vi "scale raw data.vi"(6 "ch3":waveform(dbl), 7 "Signal scaling control":T2={"Iin ripple gain"=13.333, "Iout ripple gain"=13.333, "Iout 60Hz gain "=14.286, "Vout 60Hz gain "=20.0, "Iin ripple offest"=0.0, "Iout ripple offset"=0.0, "Iout 60Hz offset"=0.0, "Vout 60Hz offset"=0.0}, 8 "error in (no error)":errorcluster, 9 "ch2":waveform(dbl), 10 "ch1":waveform(dbl), 11 "ch0":waveform(dbl)) -> (0 "error out":errorcluster, 3 "output channels WF":T1, 4 "Signal scaling control (dup out)":T2={"Iin ripple gain"=13.333, "Iout ripple gain"=13.333, "Iout 60Hz gain "=14.286, "Vout 60Hz gain "=20.0, "Iin ripple offest"=0.0, "Iout ripple offset"=0.0, "Iout 60Hz offset"=0.0, "Vout 60Hz offset"=0.0})   [LabVIEW 2019, in "Main.lvclass"]
doc: "Developed by Kevin Thompson\nkevin@thompsonengineering.net\n\nCopyright 2020\nThompson Engineering, LLC"
uses:
  Main.lvclass
  DataTypes/Gain control.ctl
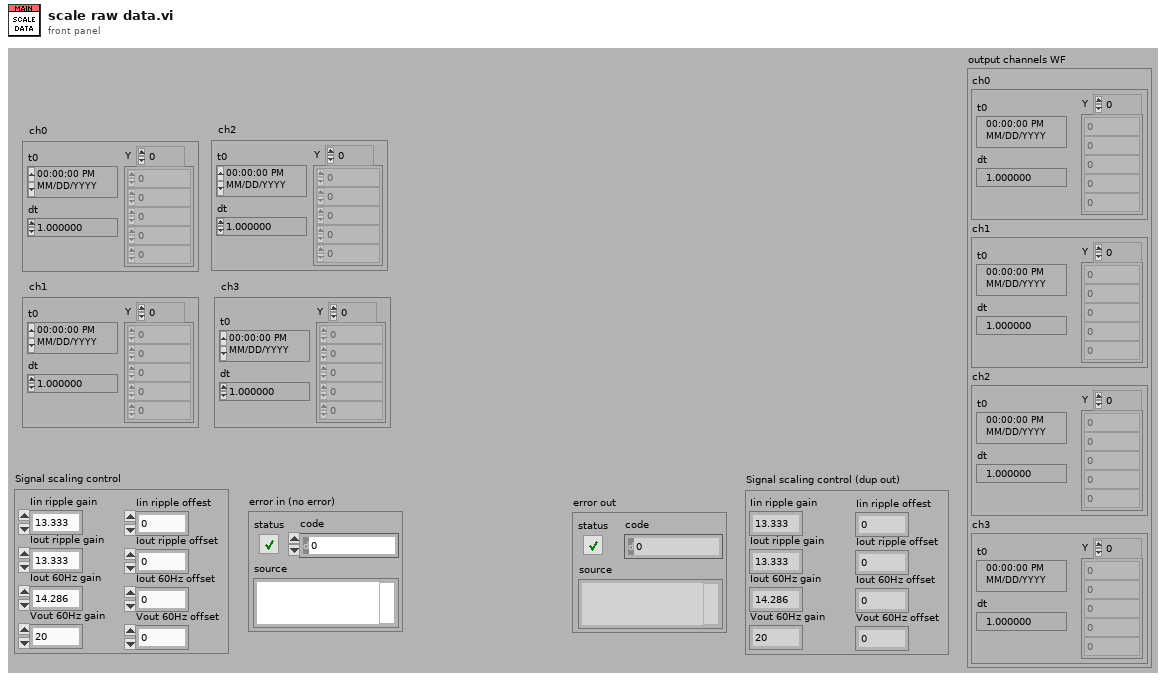
[diagram p1: front panel]
types:
  T1 = cluster{"ch0":waveform(dbl), "ch1":waveform(dbl), "ch2":waveform(dbl), "ch3":waveform(dbl)}
  T2 = typedef "Main.lvclass/Gain control.ctl" = cluster{"Iin ripple gain":dbl, "Iout ripple gain":dbl, "Iout 60Hz gain ":dbl, "Vout 60Hz gain ":dbl, "Iin ripple offest":dbl, "Iout ripple offset":dbl, "Iout 60Hz offset":dbl, "Vout 60Hz offset":dbl}
  T3 = cluster{"waveform out":waveform(dbl), "waveform out":waveform(dbl), "waveform out":waveform(dbl), "waveform out":waveform(dbl)}
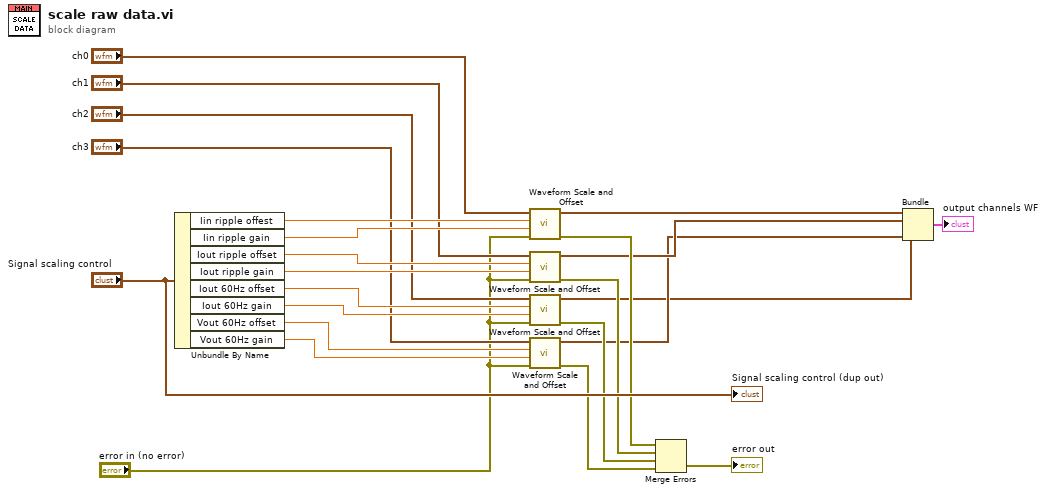
[diagram p0: block diagram]
diagram:
  n1 = Unbundle By Name("Signal scaling control") -> ("Iin ripple offest"=w24:dbl, "Iin ripple gain"=w23:dbl, "Iout ripple offset"=w22:dbl, "Iout ripple gain"=w21:dbl, "Iout 60Hz offset"=w20:dbl, "Iout 60Hz gain"=w19:dbl, "Vout 60Hz offset"=w18:dbl, "Vout 60Hz gain"=w17:dbl)
  n2 = call <vilib>:"Waveform Scale and Offset.vi"("error in (no error)"="error in (no error)", "scale"=w23, "offset"=w24, "waveform in"="ch0") -> ("error out"=w10:errorcluster, "waveform out"=w5:waveform(dbl))  [unwired: 6 in]
  n3 = call <vilib>:"Waveform Scale and Offset.vi"("error in (no error)"="error in (no error)", "scale"=w21, "offset"=w22, "waveform in"="ch1") -> ("error out"=w9:errorcluster, "waveform out"=w4:waveform(dbl))  [unwired: 6 in]
  n4 = call <vilib>:"Waveform Scale and Offset.vi"("error in (no error)"="error in (no error)", "scale"=w19, "offset"=w20, "waveform in"="ch2") -> ("error out"=w8:errorcluster, "waveform out"=w2:waveform(dbl))  [unwired: 6 in]
  n5 = call <vilib>:"Waveform Scale and Offset.vi"("error in (no error)"="error in (no error)", "scale"=w17, "offset"=w18, "waveform in"="ch3") -> ("error out"=w7:errorcluster, "waveform out"=w3:waveform(dbl))  [unwired: 6 in]
  n6 = Merge Errors(w10, w9, w8, w7) -> (→"error out":errorcluster)
  n7 = Bundle("waveform out"=w5, "waveform out"=w4, "waveform out"=w2, "waveform out"=w3) -> (→"output channels WF":T3)  [unwired: 1 in]
  "Signal scaling control (dup out)" <- "Signal scaling control"
